vi "Get Section Data.vi"(8 "error in":errorcluster, 11 "Section Ref in":refnum<data-value>) -> (0 "error out":errorcluster, 2 "Section Data":T1, 3 "Section Ref out":refnum<data-value>)   [LabVIEW 2024, in "Config File Parser.lvlib" / "Section.lvclass"]
uses:
  Section.lvclass
  Section.lvclass/Section.ctl
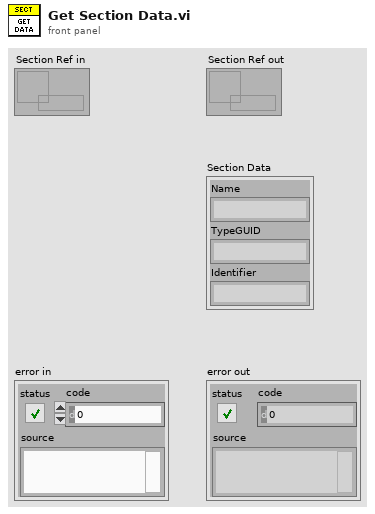
[diagram p1: front panel]
types:
  T1 = cluster{"Name":string, "TypeGUID":string, "Identifier":string}
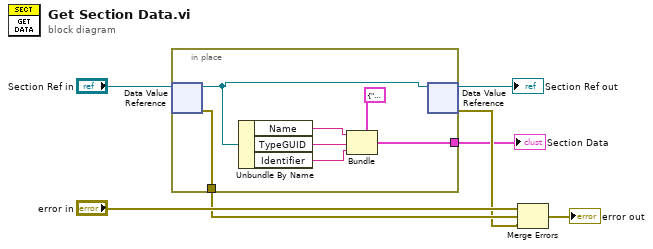
[diagram p0: block diagram]
diagram:
  n1 = in-place "In Place Element Structure" {
    in-place-border: [w14] -> w6
    in-place-border: [w8] -> w3
    n2 = in-place-dvr #1("Section Ref in") -> (w9:refnum<class "Section.lvclass">, w14:errorcluster)
    n3 = Unbundle By Name(w9) -> ("Name"=w12:string, "TypeGUID"=w11:string, "Identifier"=w10:string)
    n4 = Bundle(cluster=T1 {"Name"="", "TypeGUID"="", "Identifier"=""}, "Name"=w12, "TypeGUID"=w11, "Identifier"=w10) -> (w8:T1)
    n5 = in-place-dvr #1(w9) -> (→"Section Ref out":refnum<data-value>, w5:errorcluster)
  }
  "Section Data" <- w3
  n6 = Merge Errors("error in", w6, w5) -> (→"error out":errorcluster)
